vi "Store Current Bounds.vi"(8 "error in (no error)":errorcluster, 11 "GVIWebProcessorApp in":refnum<class "GVIWebProcessorApp.lvclass">) -> (0 "error out":errorcluster, 3 "GVIWebProcessorApp out":refnum<class "GVIWebProcessorApp.lvclass">)   [LabVIEW 2020, in "PicoG-Processor.lvlib" / "GVIWebProcessorApp.lvclass"]
uses:
  GVIWebProcessorApp.lvclass
  GVIWebProcessorApp.lvclass/GVIWebProcessorApp.ctl
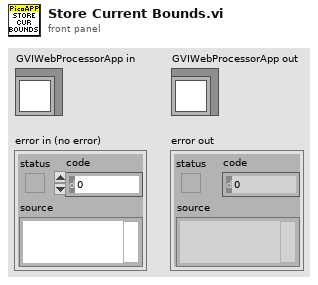
[diagram p1: front panel]
types:
  T1 = typedef "PicoG-Processor.lvlib/GVIWebProcessorApp.lvclass/Ref Data.ctl" = cluster{"hWnd":i32, "UI Refs":T2, "Collapsed":bool, "Async Anim Ref":refnum<vi>, "Expanded Bounds":T3, "Expanding":bool, "Collapsing":bool}
  T2 = typedef "PicoG-Processor.lvlib/GVIWebProcessorApp.lvclass/UI Refs.ctl" = cluster{"Main Window":refnum<vi>, "List Panel":refnum<vi>, "H Splitter":refnum<vi>, "V Splitter":refnum<vi>, "Open Project":refnum<vi>, "Project Name":refnum<vi>}
  T3 = typedef "LVRectTypeDef.ctl" = cluster{"Left":i16, "Top":i16, "Right":i16, "Bottom":i16}
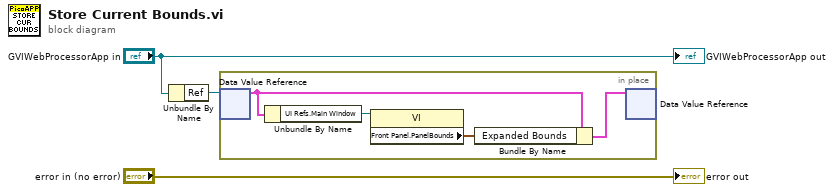
[diagram p0: block diagram]
diagram:
  n1 = Unbundle By Name("GVIWebProcessorApp in") -> ("Ref"=w1:refnum<data-value>)
  n2 = in-place {
    n3 = in-place-dvr #1(w1) -> (w6:T1)  [unwired: 1 out]
    n4 = Unbundle By Name(w6) -> ("UI Refs.Main Window"=w7:refnum<vi>)
    n5 = property class="VI"(reference=w7) -> ("Front Panel.PanelBounds"=w5:T3)  [unwired: 1 in, 2 out]
    n6 = Bundle By Name(cluster=w6, "Expanded Bounds"=w5) -> (w4:T1)
    n7 = in-place-dvr #1(w4) -> ()  [unwired: 2 out]
  }
  "error out" <- "error in (no error)"
  "GVIWebProcessorApp out" <- "GVIWebProcessorApp in"
